vi "Send Command.vi"(8 "error in (no error)":errorcluster, 11 "UI Command Manager in":refnum<class "UI Command Manager.lvclass">) -> (0 "error out":errorcluster, 3 "UI Command Manager out":refnum<class "UI Command Manager.lvclass">)   [LabVIEW 2011, in "UI Command Manager.lvclass"]
uses:
  UI Command Manager.lvclass
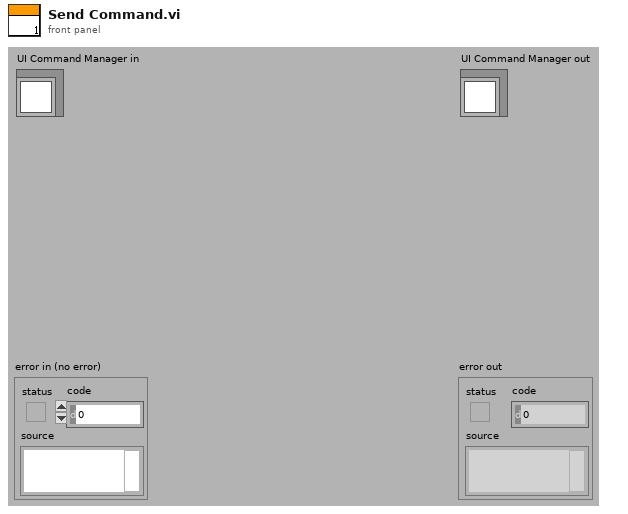
[diagram p1: front panel]
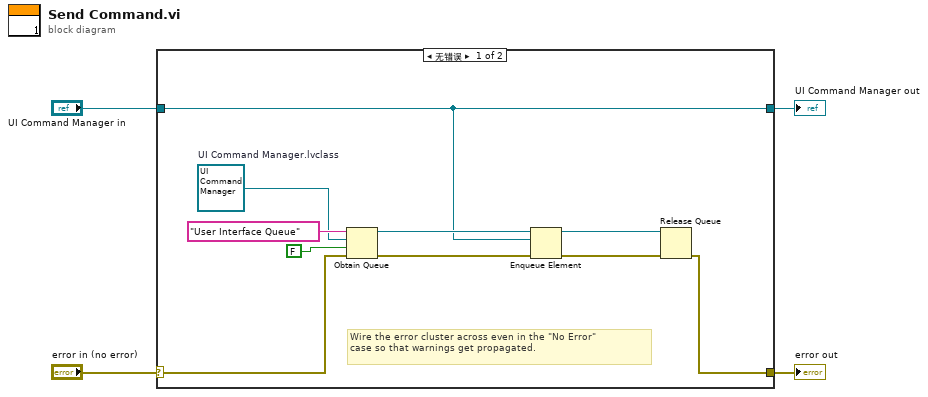
[diagram p0: block diagram]
diagram:
  n1 = case shown="无错误" "error in (no error)" {
    selector: "error in (no error)" -> [w9 w16]
    tunnel: [w5 w16] -> w3
    tunnel: [w10 w15] -> w1
    tunnel: "UI Command Manager in" -> [w10 w15]
    frame No Error {
      w13 = refnum<class "UI Command Manager.lvclass"> refnum  # UI Command Manager.lvclass
      # "Wire the error cluster across even in the \"No Error\"\ncase so that warnings get propagated."
      n2 = Obtain Queue(name (unnamed)="User Interface Queue", element data type=w13, create if not found? (T)=FALSE, error in (no error)=w9) -> (queue out=w12:refnum<queue>, error out=w11:errorcluster)  [unwired: 1 in, 1 out]
      n3 = Enqueue Element(queue=w12, element=w10, error in (no error)=w11) -> (queue out=w6:refnum<queue>, error out=w7:errorcluster)  [unwired: 1 in, 1 out]
      n4 = Release Queue(queue=w6, error in (no error)=w7) -> (error out=w5:errorcluster)  [unwired: 1 in, 2 out]
    }
    frame Error {
    }
  }
  "error out" <- w3
  "UI Command Manager out" <- w1
